vi "Dispense.vi"(0 "reference in":refnum<class "Sold State.lvclass">, 5 "error in (no error)":errorcluster) -> (14 "reference out":refnum<class "Sold State.lvclass">, 19 "error out":errorcluster)   [LabVIEW 2013, in "Sold State.lvclass"]
uses:
  Sold State.lvclass
  Gum Machine_class/Gum Machine.lvclass
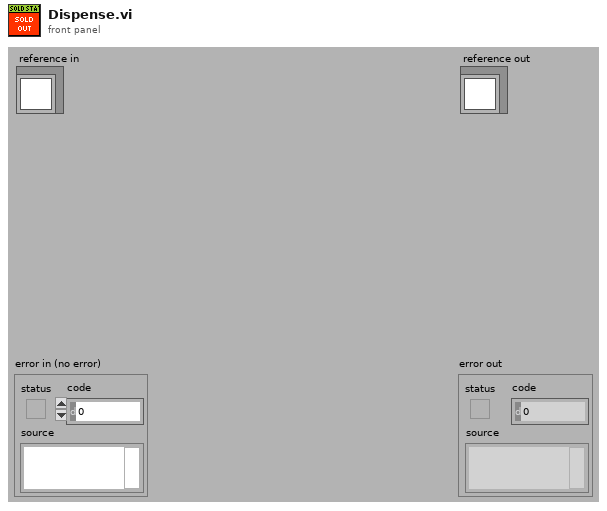
[diagram p1: front panel]
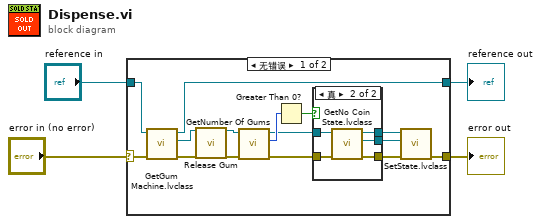
[diagram p0: block diagram]
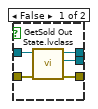
[diagram p2: hidden frame]
diagram:
  n1 = case shown="无错误" "error in (no error)" {
    selector: "error in (no error)" -> [w17 w31]
    tunnel: [w5 w31] -> w3
    tunnel: [w18 w30] -> w1
    tunnel: "reference in" -> [w19 w30]
    frame No Error {
      n2 = call-dynamic "GetGum Machine.lvclass.vi"("error in (no error)"=w17, "reference in"=w19) -> ("error out"=w16:errorcluster, "Gum Machine.lvclass"=w14:refnum<class "Gum Machine.lvclass">, "reference out"=w18:refnum<class "Sold State.lvclass">)  [unwired: 7 in]
      n3 = call-dynamic "Release Gum.vi"("reference in"=w14, "error in (no error)"=w16) -> ("reference out"=w13:refnum<class "Gum Machine.lvclass">, "error out"=w15:errorcluster)  [unwired: 16 in]
      n4 = call-dynamic "GetNumber Of Gums.vi"("error in (no error)"=w15, "reference in"=w13) -> ("error out"=w10:errorcluster, "Number Of Gums"=w12:u32, "reference out"=w11:refnum<class "Gum Machine.lvclass">)  [unwired: 7 in]
      n5 = Greater Than 0?(x=w12) -> (x > 0?=w9:bool)
      n6 = case shown="真" w9 {
        tunnel: w11 -> [w24 w29]
        tunnel: w10 -> [w23 w28]
        tunnel: [w21 w27] -> w8
        tunnel: [w22 w26] -> w7
        tunnel: [w20 w25] -> w6
        frame False {
          n7 = call-dynamic "GetSold Out State.lvclass.vi"("error in (no error)"=w23, "reference in"=w24) -> ("error out"=w20:errorcluster, "Sold Out State.lvclass"=w21:refnum<class "Sold Out State.lvclass">, "reference out"=w22:refnum<class "Gum Machine.lvclass">)  [unwired: 7 in]
        }
        frame True {
          n8 = call-dynamic "GetNo Coin State.lvclass.vi"("error in (no error)"=w28, "reference in"=w29) -> ("error out"=w25:errorcluster, "No Coin State.lvclass"=w27:refnum<class "No Coin State.lvclass">, "reference out"=w26:refnum<class "Gum Machine.lvclass">)  [unwired: 7 in]
        }
      }
      n9 = call-dynamic "SetState.lvclass.vi"("error in (no error)"=w6, "State.lvclass"=w8, "reference in"=w7) -> ("error out"=w5:errorcluster)  [unwired: 7 in, 1 out]
    }
    frame Error {
    }
  }
  "error out" <- w3
  "reference out" <- w1
